vi "Cleanup Measurement.vi"(8 "error in":errorcluster, 10 "measurement plug-in name":string, 11 "project path":path) -> (0 "error out":errorcluster)   [LabVIEW 2021, in "Converter.lvlib"]
uses:
  Converter.lvlib
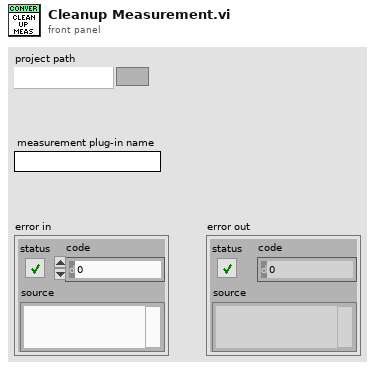
[diagram p1: front panel]
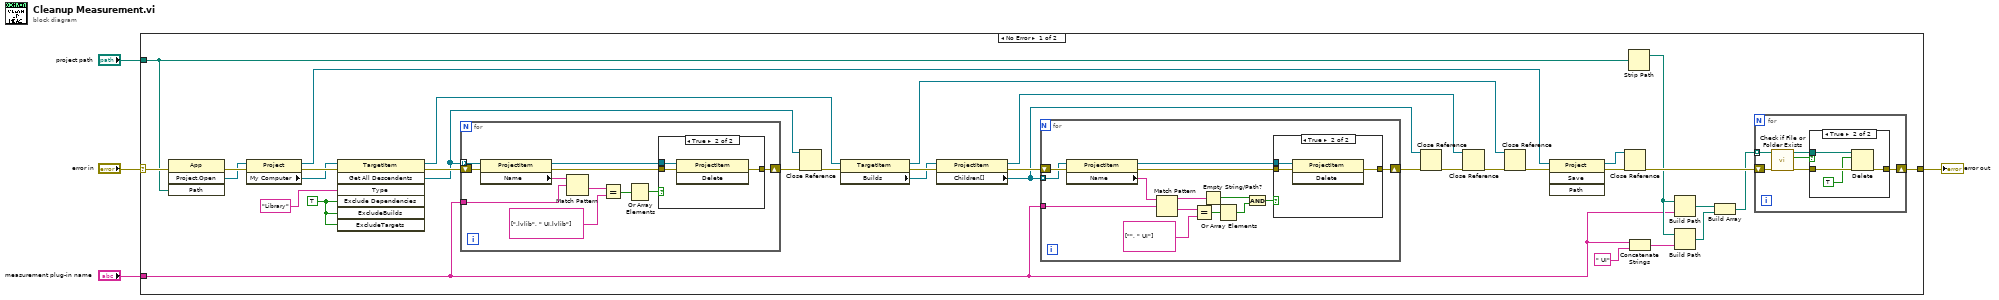
[diagram p0: block diagram]
diagram:
  n1 = case shown="No Error" "error in" {
    selector: "error in" -> [w35 w84]
    tunnel: "measurement plug-in name" -> [w6 _]
    tunnel: [w11 w84] -> w1
    tunnel: "project path" -> [w5 _]
    frame No Error {
      w20 = TRUE ("ExcludeDependencies")
      n2 = invoke class="App" method="Project.Open"(error in=w35, "Path"=w5) -> (error out=w36:errorcluster, "Project:Open"=w18:refnum<vi>)  [unwired: 2 in, 2 out]
      n3 = property class="Project"(reference=w18, error in=w36) -> (reference out=w21:refnum<vi>, error out=w37:errorcluster, "My Computer"=w31:refnum<vi>)
      n4 = invoke class="TargetItem" method="Get All Descendents"(reference=w31, error in=w37, "Type"="Library", "Exclude Dependencies"=w20, "ExcludeBuilds"=w20, "ExcludeTargets"=w20) -> (reference out=w30:refnum<vi>, error out=w38:errorcluster, "All Descendents"=w33:refnum<vi>[])  [unwired: 1 in, 4 out]
      n5 = for {
        shift-right: [w73] -> w39
        shift-left: w38 -> [w79]
        tunnel: w33 -> [w78] mode=indexing
        tunnel: w6 -> [w70]
        n6 = property class="ProjectItem"(reference=w78, error in=w79) -> (reference out=w72:refnum<vi>, error out=w74:errorcluster, "Name"=w77:string)
        n7 = Match Pattern(string=w77, regular expression=w70) -> (after substring=w76:string)  [unwired: 1 in, 3 out]
        n8 = Equal?(x=w76, y=string[] [".lvlib", " UI.lvlib"]) -> (x = y?=w69:bool[])
        n9 = Or Array Elements(Boolean array=w69) -> (logical OR=w71:bool)
        n10 = case shown="True" w71 {
          tunnel: w74 -> [w80 w83]
          tunnel: [w80 w82] -> w73
          tunnel: w72 -> [_ w81]
          frame False {
          }
          frame True {
            n11 = invoke class="ProjectItem" method="Delete"(reference=w81, error in=w83) -> (error out=w82:errorcluster)  [unwired: 1 in, 2 out]
          }
        }
      }
      n12 = Close Reference(reference=w33, error in (no error)=w39) -> (error out=w32:errorcluster)
      n13 = property class="TargetItem"(reference=w30, error in=w32) -> (reference out=w24:refnum<vi>, error out=w25:errorcluster, "Builds"=w23:refnum<vi>)
      n14 = property class="ProjectItem"(reference=w23, error in=w25) -> (reference out=w22:refnum<vi>, error out=w29:errorcluster, "Children[]"=w26:refnum<vi>[])
      n15 = for {
        shift-right: [w61] -> w28
        shift-left: w29 -> [w64]
        tunnel: w26 -> [w62] mode=indexing
        tunnel: w6 -> [w58]
        n16 = property class="ProjectItem"(reference=w62, error in=w64) -> (reference out=w60:refnum<vi>, error out=w63:errorcluster, "Name"=w59:string)
        n17 = Match Pattern(string=w59, regular expression=w58) -> (before substring=w55:string, after substring=w54:string)  [unwired: 1 in, 2 out]
        n18 = Equal?(x=w54, y=string[] ["", " UI"]) -> (x = y?=w57:bool[])
        n19 = Empty String/Path?(string/path=w55) -> (empty?=w51:bool)
        n20 = Or Array Elements(Boolean array=w57) -> (logical OR=w52:bool)
        n21 = And(x=w51, y=w52) -> (x .and. y?=w56:bool)
        n22 = case shown="True" w56 {
          tunnel: w63 -> [w65 w68]
          tunnel: [w65 w67] -> w61
          tunnel: w60 -> [_ w66]
          frame False {
          }
          frame True {
            n23 = invoke class="ProjectItem" method="Delete"(reference=w66, error in=w68) -> (error out=w67:errorcluster)  [unwired: 1 in, 2 out]
          }
        }
      }
      n24 = Close Reference(reference=w26, error in (no error)=w28) -> (error out=w27:errorcluster)
      n25 = Close Reference(reference=w22, error in (no error)=w27) -> (error out=w17:errorcluster)
      n26 = Close Reference(reference=w24, error in (no error)=w17) -> (error out=w16:errorcluster)
      n27 = invoke class="Project" method="Save"(reference=w21, error in=w16) -> (reference out=w13:refnum<vi>, error out=w15:errorcluster)  [unwired: 2 in, 2 out]
      n28 = Close Reference(reference=w13, error in (no error)=w15) -> (error out=w14:errorcluster)
      n29 = Strip Path(path=w5) -> (stripped path=w12:path)  [unwired: 1 out]
      n30 = Concatenate Strings(w6, " UI" ("string")) -> (w34:string)
      n31 = Build Path(base path=w12, name or relative path=w6) -> (appended path=w8:path)
      n32 = Build Path(base path=w12, name or relative path=w34) -> (appended path=w9:path)
      n33 = Build Array(w8, w9) -> (w7:path[])
      n34 = for {
        shift-right: [w44] -> w11
        shift-left: w14 -> [w45]
        tunnel: w7 -> [w40] mode=indexing
        n35 = call <vilib>:"Check if File or Folder Exists.vi"("error in (no error)"=w45, "path"=w40) -> ("error out"=w43:errorcluster, "file or folder exists?"=w42:bool, "dup path"=w41:path)  [unwired: 7 in]
        n36 = case shown="True" w42 {
          tunnel: w43 -> [w46 w50]
          tunnel: [w46 w49] -> w44
          tunnel: w41 -> [_ w48]
          frame False {
          }
          frame True {
            n37 = Delete(path (use dialog)=w48, entire hierarchy (F)=TRUE, error in=w50) -> (error out=w49:errorcluster)  [unwired: 2 in, 2 out]
          }
        }
      }
    }
    frame Error {
    }
  }
  "error out" <- w1
